vi "字符键盘.vi"(11 "Old String":string) -> (3 "String":string)   [LabVIEW 2016, in "斯坦道总氮.lvlib"]
panel:
  in  "^":bool
  in  "$":bool
  in  "!":bool
  in  "~":bool
  in  "%":bool
  in  "&":bool
  in  "@":bool
  in  "_":bool
  in  "#":bool
  in  "大小写":bool
  in  "Z":bool
  in  "Y":bool
  in  "X":bool
  in  "W":bool
  in  "V":bool
  in  "U":bool
  in  "T":bool
  in  "S":bool
  in  "R":bool
  in  "Q":bool
  in  "P":bool
  in  "O":bool
  in  "N":bool
  in  "M":bool
  in  "L":bool
  in  "K":bool
  in  "J":bool
  in  "I":bool
  in  "H":bool
  in  "G":bool
  in  "F":bool
  in  "E":bool
  in  "D":bool
  in  "C":bool
  in  "B":bool
  in  "A":bool
  in  ",":bool
  in  "Cancel":bool
  in  "OK":bool
  in  "Clear":bool
  in  "BackSpace":bool
  in  "Point":bool
  in  "Zero":bool
  in  "Nine":bool
  in  "Eight":bool
  in  "Seven":bool
  in  "Six":bool
  in  "Five":bool
  in  "Four":bool
  in  "Three":bool
  in  "Two":bool
  in  "One":bool
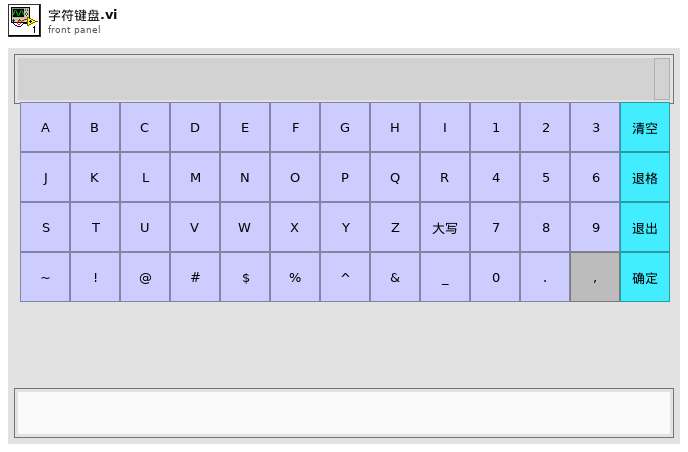
[diagram p1: front panel]
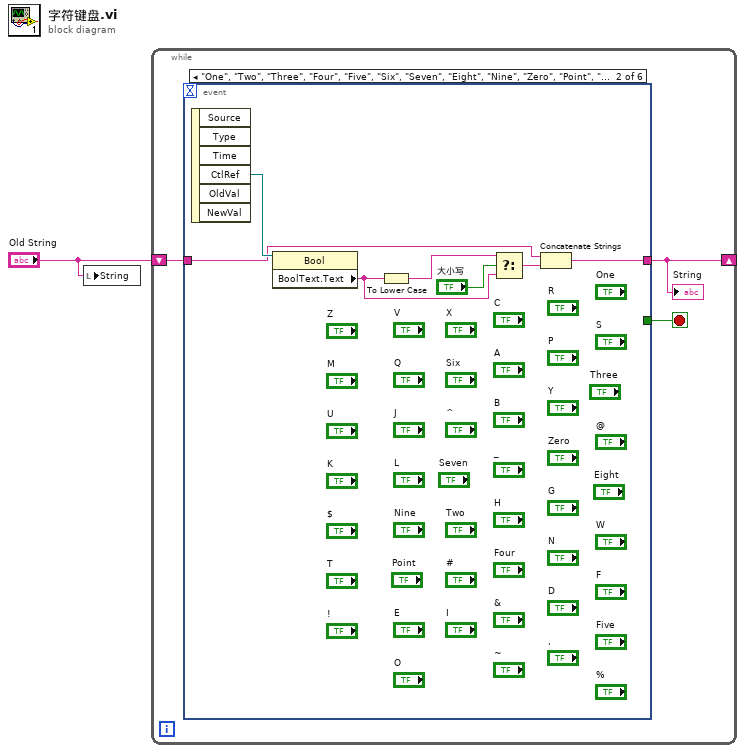
[diagram p0: block diagram]
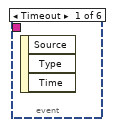
[diagram p2: hidden frame]
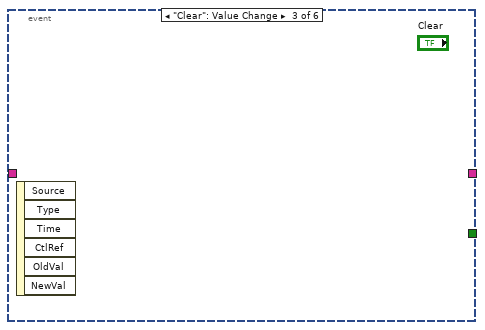
[diagram p3: hidden frame]
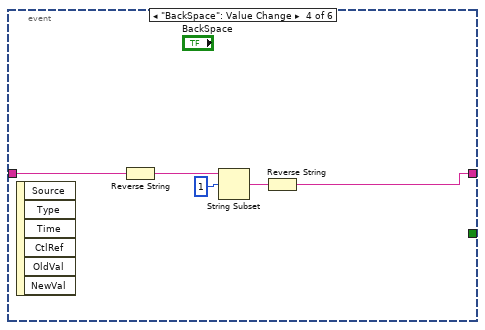
[diagram p4: hidden frame]
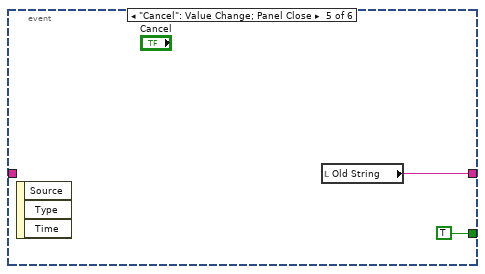
[diagram p5: hidden frame]
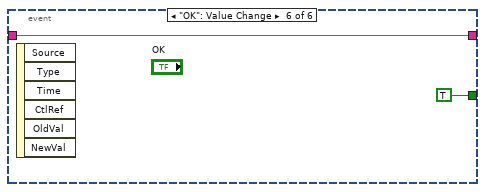
[diagram p6: hidden frame]
diagram:
  n1 = local write "String"("Old String") -> ()
  n2 = while {
    shift-right: [w3] -> _
    shift-left: "Old String" -> [w4]
    stop <- w2 stop-if-true
    n3 = event shown="[1] \"One\", \"Two\", \"Three\", \"Four\", \"Five\", \"Six\", \"Seven\", \"Eight\", \"Nine\", \"Zero\", \"Point\", \"A\", \"B\", \"C\", \"D\", \"E\", \"F\", \"G\", \"H\", \"I\", \"J\", \"K\", \"L\", \"M\", \"N\", \"O\", \"P\", \"Q\", \"R\", \"S\", \"T\", \"U\", \"V\", \"W\", \"X\", \"Y\", \"Z\", \"#\", \"_\", \"@\", \"&\", \"%\", \"~\", \"!\", \"$\", \"^\", \",\": Value Change" {
      selector: _ -> [_ _ _ _ _ _]
      dyn-events: _ -> [_ _ _ _ _ _]
      timeout: _ -> [_ _ _ _ _ _]
      tunnel: w4 -> [_ w10 _ w15 _ w20]
      tunnel: [_ w9 _ w12 w18 w20] -> w3
      tunnel: [_ _ _ _ TRUE TRUE] -> w2
      event Timeout {
        n4 = event-data() -> ()  [unwired: 1 in, 3 out]
      }
      event "One", "Two", "Three", "Four", "Five", "Six", "Seven", "Eight", "Nine", "Zero", "Point", "A", "B", "C", "D", "E", "F", "G", "H", "I", "J", "K", "L", "M", "N", "O", "P", "Q", "R", "S", "T", "U", "V", "W", "X", "Y", "Z", "#", "_", "@", "&", "%", "~", "!", "$", "^", ",": Value Change {
        n5 = event-data() -> ("CtlRef"=w11:refnum<vi>)  [unwired: 1 in, 5 out]
        n6 = property class="Bool"(reference=w11) -> ("BoolText.Text"=w5:string)  [unwired: 1 in, 2 out]
        n7 = To Lower Case(string=w5) -> (all lower case string=w6:string)
        n8 = Select(t=w6, s="大小写", f=w5) -> (s? t:f=w7:string)
        n9 = Concatenate Strings(w10, w7) -> (w9:string)
      }
      event "Clear": Value Change {
        n10 = event-data() -> ()  [unwired: 1 in, 6 out]
      }
      event "BackSpace": Value Change {
        n11 = event-data() -> ()  [unwired: 1 in, 6 out]
        n12 = Reverse String(1:w15) -> (0:w14:string)
        n13 = String Subset(string=w14, offset (0)=1 ("偏移量(0)")) -> (substring=w13:string)  [unwired: 1 in]
        n14 = Reverse String(1:w13) -> (0:w12:string)
      }
      event "Cancel": Value Change; Panel Close {
        n15 = event-data() -> ()  [unwired: 1 in, 3 out]
        n16 = local read "Old String"() -> (w18:string)
      }
      event "OK": Value Change {
        n17 = event-data() -> ()  [unwired: 1 in, 6 out]
      }
    }
    "String" <- w3
  }
